vi "host_chunk_dvr.vi"() -> ()   [LabVIEW 2020]
doc: "This example demonstrates how to continuously acquire buffered voltage measurements using a DAQmx device.\n\nFor instructions on how to connect your signals to the DAQ device, refer to your device documentation."
uses:
  <vilib>/DAQmx/read.llb/DAQmx Read (Analog Wfm 1Chan NSamp).vi
  <vilib>/DAQmx/create/channels.llb/DAQmx Create Channel (AI-Voltage-Basic).vi
  <vilib>/DAQmx/configure/timing.llb/DAQmx Timing (Sample Clock).vi
  <vilib>/FPGAPlugInAG/cRIO-9040/niLvFpga_Open_cRIO-9040.vi
  <vilib>/rvi/interface/common/dynamic/niFpgaDynamicAddResources.vi
  <vilib>/Utility/error.llb/Error Cluster From Error Code.vi
  <vilib>/rvi/errors/niLvFpgaAdjustHostInterfaceError.vi
  <vilib>/FPGAPlugInAG/Dynamic/niLvFpga_Run_Dynamic.vi
  <vilib>/RVI Host/nirviSupport.llb/nirviErrorClusterFromErrorCode.vi
  <vilib>/DAQmx/miscellaneous.llb/DAQmx Fill In Error Info.vi
  <vilib>/FPGAPlugInAG/Dynamic/niLvFpga_Close_Dynamic.vi
  <vilib>/rvi/interface/nirviOpenFPGA/nirviOpenFPGA.xnode
  FPGA Bitfiles/testDMA_9040_chunk_v1001.lvbitx
  <vilib>/rvi/interface/nirviReadWriteControl/nirviReadWriteControl.xnode
  <vilib>/rvi/interface/nirviMethod/nirviMethod.xnode
  <vilib>/rvi/interface/nirviCloseFPGA/nirviCloseFPGA.xnode
  <resource>/objmgr/daqmx.rc
  <vilib>/rvi/interface/Simulation/niFpgaSimulationCallBeginRW.vi
  <vilib>/rvi/errors/niLvFpgaMergeErrorWithErrorCode.vi
  NiFpgaLv.dll
  <vilib>/rvi/interface/nirviMethod/StockFPGA_InlinedMethodWaitForSingleIRQ.vi
  <vilib>/FPGAPlugInAG/Dynamic/niLvFpga_WaitOnIrq_Dynamic.vi
  <vilib>/FPGAPlugInAG/Dynamic/niLvFpga_AcknowledgeIrq_Dynamic.vi
  <vilib>/FPGAPlugInAG/Dynamic/niLvFpga_AcquireWriteRegionFifo_Dynamic.vi
  <vilib>/FPGAPlugInAG/Dynamic/niLvFpga_AcquireReadRegionFifo_Dynamic.vi
panel:
  out "dma read time uS":u32
  out "AvailSampPerChan":u32
  out "write DMA timeout count":i16
  out "uS elapsed":cluster{u32, u32}(graph)
  out "Timed Out":bool
  out "error out":errorcluster
  in  "Stop":bool
  out "Waveform Graph":dbl[][](graph)
  in  "Number of Samples":i32=100
  in  "Sample Rate":dbl=1000.0
  in  "Sample Clock Source":tag="OnboardClock"
  in  "Terminal Configuration":i32(ring)=-1 items=["default"=-1, "RSE"=10083, "NRSE"=10078, "Differential"=10106, "Pseudodifferential"=12529]
  in  "Max Voltage":dbl=5.0
  in  "Min Voltage":dbl=-5.0
  in  "Physical Channel":tag="Dev1/ai0"
  out "Actual Sample Rate":dbl=1000.0 format="%0.2f"
  # "Channel Settings"
  # "Acquired Data"
  # "Timing Settings"
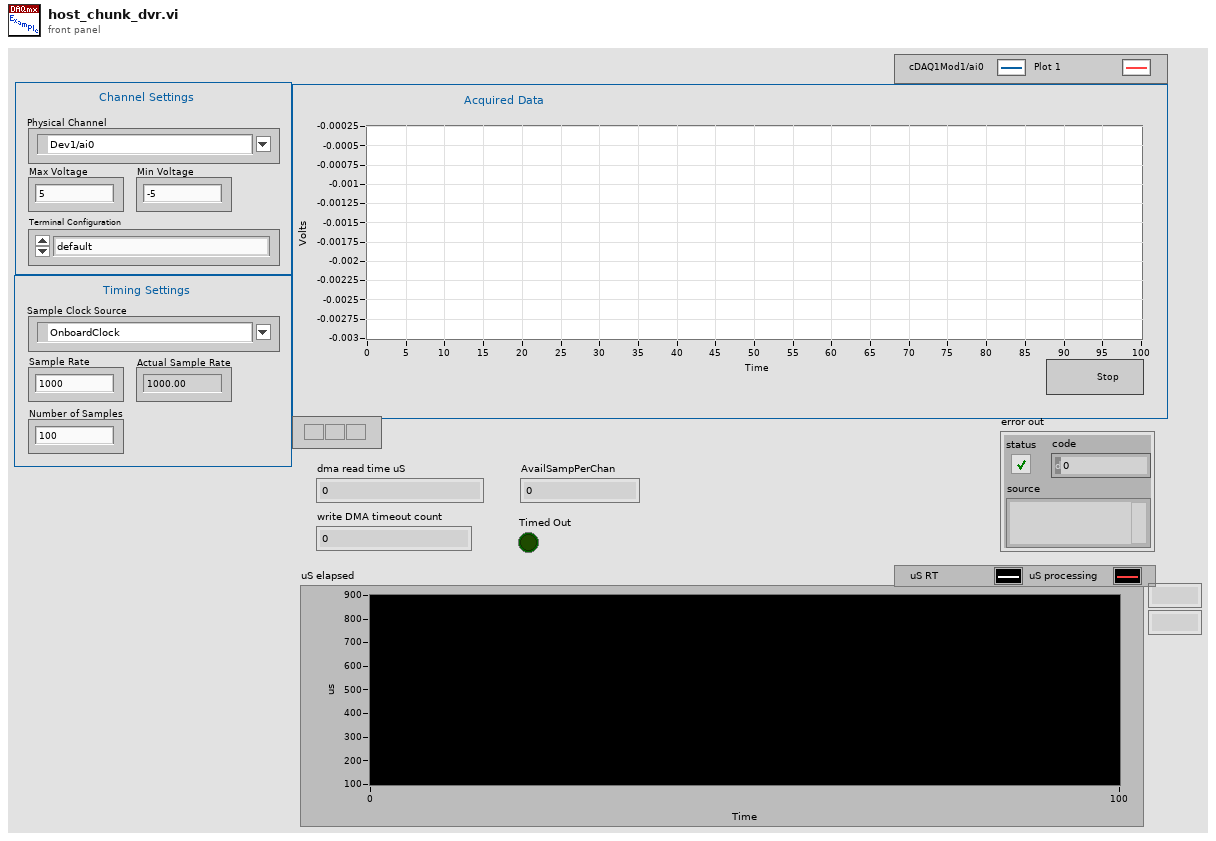
[diagram p1: front panel]
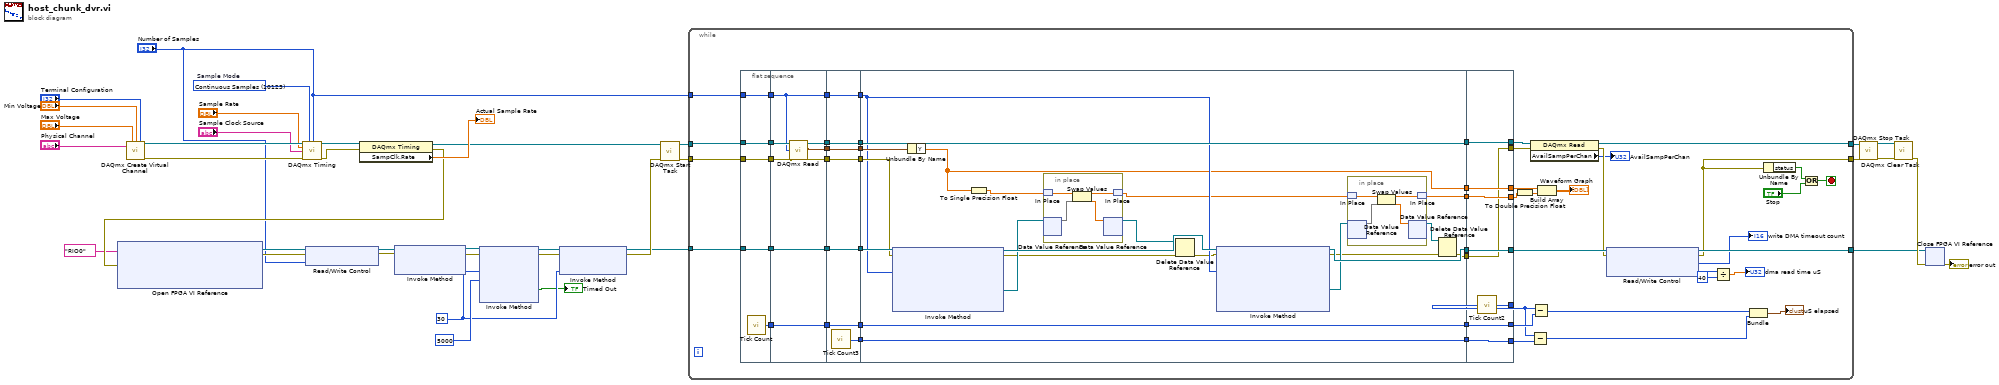
[diagram p0: block diagram]
diagram:
  w5 = u8 30 ("IRQ Number (0)")
  w36 = 10123 items=["Finite Samples"=10178, "Continuous Samples"=10123, "Hardware Timed Single Point"=12522]  # Sample Mode
  n1 = call-poly <vilib>:"DAQmx Create Virtual Channel.vi"("maximum value"="Max Voltage", "minimum value"="Min Voltage", "input terminal configuration"="Terminal Configuration", "physical channels"="Physical Channel") -> ("task out"=w34:refnum<k21>, "error out"=w35:errorcluster)  [unwired: 10 in]
  n2 = call-poly <vilib>:"DAQmx Timing.vi"("task/channels in"=w34, "sample mode"=w36, "samples per channel"="Number of Samples", "rate"="Sample Rate", "source"="Sample Clock Source", "error in"=w35) -> ("task out"=w38:refnum<k21>, "error out"=w37:errorcluster)  [unwired: 8 in]
  n3 = property class="DAQmx Timing"(reference=w38, error in=w37) -> (reference out=w17:refnum<k21>, error out=w18:errorcluster, "SampClk.Rate"=→"Actual Sample Rate":dbl)
  n4 = xnode "Open FPGA VI Reference"("error in"=w18, "resource name"=tag "RIO0") -> ("FPGA VI Reference Out"=w15:refnum<k20>, "error out"=w16:errorcluster)
  n5 = xnode "Read/Write Control"("FPGA VI Reference In"=w15, "error in"=w16, "number of samples"="Number of Samples") -> ("FPGA VI Reference Out"=w12:refnum<k20>, "error out"=w11:errorcluster)
  n6 = xnode "Invoke Method"("FPGA VI Reference In"=w12, "error in"=w11) -> ("FPGA VI Reference Out"=w10:refnum<k20>, "error out"=w9:errorcluster)  [unwired: 1 in]
  n7 = xnode "Invoke Method"("FPGA VI Reference In"=w10, "error in"=w9, "IRQ Number(s)"=w5, "Timeout (ms)"=5000) -> ("FPGA VI Reference Out"=w8:refnum<k20>, "error out"=w7:errorcluster, "Timed Out"=→"Timed Out":bool)  [unwired: 1 out]
  n8 = xnode "Invoke Method"("FPGA VI Reference In"=w8, "error in"=w7, "IRQ Number(s)"=w5) -> ("FPGA VI Reference Out"=w2:refnum<k20>, "error out"=w3:errorcluster)
  n9 = call <vilib>:"DAQmx Start Task.vi"("task/channels in"=w17, "error in"=w3) -> ("task out"=w33:refnum<k21>, "error out"=w32:errorcluster)  [unwired: 12 in]
  n10 = while {
    tunnel: w33 -> [w92]
    tunnel: w32 -> [w87]
    tunnel: [w72] -> w24
    tunnel: [w75] -> w23
    tunnel: "Number of Samples" -> [w61]
    tunnel: w2 -> [w86]
    tunnel: [w76] -> w1
    stop <- w88 stop-if-true
    n11 = flat-sequence {
      tunnel: w92 -> [w97]
      tunnel: [w97] -> w66
      tunnel: [w96] -> w65
      tunnel: w87 -> [w96]
      tunnel: [w95] -> w64
      tunnel: w86 -> [w95]
      tunnel: [w94] -> w63
      tunnel: [w93] -> w62
      tunnel: w61 -> [w93]
      tunnel: w66 -> [w103]
      tunnel: [w103] -> w60
      tunnel: w65 -> [w102]
      tunnel: [w102] -> w58
      tunnel: w64 -> [w101]
      tunnel: [w101] -> w56
      tunnel: w63 -> [w100]
      tunnel: [w100] -> w54
      tunnel: [w99] -> w52
      tunnel: w62 -> [w98]
      tunnel: [w98] -> w50
      tunnel: w60 -> [w110]
      tunnel: [w110] -> w59
      tunnel: w58 -> [w109]
      tunnel: [w109] -> w57
      tunnel: w56 -> [w108]
      tunnel: [w108] -> w55
      tunnel: w54 -> [w107]
      tunnel: [w107] -> w53
      tunnel: w52 -> [w106]
      tunnel: [w106] -> w51
      tunnel: w50 -> [w105]
      tunnel: [w105] -> w49
      tunnel: [w104] -> w45
      tunnel: w59 -> [w125]
      tunnel: w57 -> [w126]
      tunnel: w55 -> [w131]
      tunnel: [w125] -> w82
      tunnel: [w121] -> w81
      tunnel: [w129] -> w80
      tunnel: [w128] -> w78
      tunnel: w53 -> [w128]
      tunnel: w51 -> [w127]
      tunnel: w49 -> [w123]
      tunnel: [w124] -> w46
      tunnel: w45 -> [w124]
      tunnel: [w112] -> w43
      tunnel: [w111] -> w39
      tunnel: [w145] -> w83
      tunnel: [w146] -> w85
      tunnel: [w147] -> w91
      tunnel: w82 -> [w147]
      tunnel: w81 -> [w146]
      tunnel: w80 -> [w145]
      tunnel: [w144] -> w48
      tunnel: [w143] -> w79
      tunnel: w78 -> [w143]
      tunnel: [w142] -> w47
      tunnel: w46 -> [w142]
      tunnel: [w141] -> w41
      tunnel: w43 -> [w141]
      tunnel: [w140] -> w40
      tunnel: w39 -> [w140]
      frame #0 {
        n12 = call "Tick Count"() -> ("Tick Count(uSec)"=w94:u32)
      }
      frame #1 {
        n13 = call-poly <vilib>:"DAQmx Read.vi"("task/channels in"=w103, "number of samples per channel"=w98, "error in"=w102) -> ("data"=w99:waveform(dbl))  [unwired: 10 in, 2 out]
      }
      frame #2 {
        n14 = call "Tick Count3"() -> ("Tick Count(uSec)"=w104:u32)
      }
      frame #3 {
        n15 = xnode "Invoke Method"("FPGA VI Reference In"=w131, "error in"=w126, "Number of Elements"=w123) -> ("FPGA VI Reference Out"=w130:refnum<k20>, "error out"=w118:errorcluster, "Write Region Reference"=w122:refnum<data-value>)  [unwired: 1 in, 2 out]
        n16 = Unbundle By Name(w127) -> ("Y"=w121:dbl[])
        n17 = To Single Precision Float(number=w121) -> (single precision float=w120:sgl[])
        n18 = in-place {
          n19 = in-place-match #1(w120) -> (w138:sgl[])
          n20 = in-place-dvr #2(w122) -> (w139:sgl[])  [unwired: 1 out]
          n21 = Swap Values(12:w138, 14:w139) -> (1:w136:sgl[], 3:w137:sgl[])  [unwired: 1 in]
          n22 = in-place-dvr #2(w137) -> (w119:refnum<data-value>)  [unwired: 1 out]
          n23 = in-place-match #1(w136) -> (w115:sgl[])
        }
        n24 = Delete Data Value Reference(data value reference=w119, error in=w118) -> (error out=w117:errorcluster)  [unwired: 1 out]
        n25 = xnode "Invoke Method"("FPGA VI Reference In"=w130, "error in"=w117, "Number of Elements"=w123) -> ("FPGA VI Reference Out"=w129:refnum<k20>, "error out"=w113:errorcluster, "Read Region Reference"=w116:refnum<data-value>)  [unwired: 1 in, 2 out]
        n26 = in-place {
          n27 = in-place-match #3(w115) -> (w134:sgl[])
          n28 = in-place-dvr #4(w116) -> (w135:sgl[])  [unwired: 1 out]
          n29 = Swap Values(12:w134, 14:w135) -> (1:w132:sgl[], 3:w133:sgl[])  [unwired: 1 in]
          n30 = in-place-dvr #4(w133) -> (w114:refnum<data-value>)  [unwired: 1 out]
          n31 = in-place-match #3(w132) -> (w112:sgl[])
        }
        n32 = Delete Data Value Reference(data value reference=w114, error in=w113) -> (error out=w111:errorcluster)  [unwired: 1 out]
      }
      frame #4 {
        n33 = call "Tick Count2"() -> ("Tick Count(uSec)"=w144:u32)
      }
    }
    n34 = To Double Precision Float(number=w41) -> (double precision float=w42:dbl[])
    n35 = property class="DAQmx Read"(reference=w91, error in=w40) -> (reference out=w72:refnum<k21>, error out=w71:errorcluster, "AvailSampPerChan"=→"AvailSampPerChan":u32)
    n36 = Subtract(x=w48, y=w47) -> (x-y=w44:u32)
    n37 = Subtract(x=w48, y=w79) -> (x-y=w77:u32)
    n38 = Build Array(w85, w42) -> (→"Waveform Graph":dbl[][])
    n39 = xnode "Read/Write Control"("FPGA VI Reference In"=w83, "error in"=w71) -> ("FPGA VI Reference Out"=w76:refnum<k20>, "error out"=w75:errorcluster, "write DMA timeout count"=→"write DMA timeout count":i16, "dma read time ticks"=w69:u32)
    n40 = Divide(x=w69, y=u32 40) -> (x/y=→"dma read time uS":dbl)
    n41 = Bundle(w77, w44) -> (→"uS elapsed":cluster{u32, u32})  [unwired: 1 in]
    n42 = Unbundle By Name(w75) -> ("status"=w89:bool)
    n43 = Or(x=w89, y="Stop") -> (x .or. y?=w88:bool)
  }
  n44 = call <vilib>:"DAQmx Stop Task.vi"("task/channels in"=w24, "error in"=w23) -> ("task out"=w21:refnum<k21>, "error out"=w22:errorcluster)  [unwired: 12 in]
  n45 = call <vilib>:"DAQmx Clear Task.vi"("task in"=w21, "error in"=w22) -> ("error out"=w20:errorcluster)  [unwired: 13 in]
  n46 = xnode "Close FPGA VI Reference"("FPGA VI Reference In"=w1, "error in"=w20) -> ("error out"=→"error out":errorcluster)
